vi "Message.vi"(0 "datain":string[](array[string])=["备注", "负载通道", "负载地址", "延时时间", "output max", "output min", "量测类型", "待测物板号"], 5 "HW CH Number":i32, 7 "Setup":string) -> (4 "REPORT INDECATE":string[][](array[string])=[["微安测试", "", "", "", ""], ["微安量测", "4", "0.000", "0.1", "NG"], ["微安量测", "4", "0.000", "0.1", "NG"], ["微安量测", "4", "0.000", "0.1", "NG"], ["微安量测", "4", "0.000", "0.1", "NG"]], 6 "ROW HEAD":string[](array[string]), 8 "PF":string[](array[string]), 10 "testData":string[](array[string]), 15 "Array":string[](array[string]))   [LabVIEW 2018]
panel:
  in  "Bar":bool
  out "结果":bool
  out "Date":string caption="messageBox"
  in  "取消":bool
  in  "确定":bool
  out "数组":bool[](array[boolean])
  # "信息提示！"
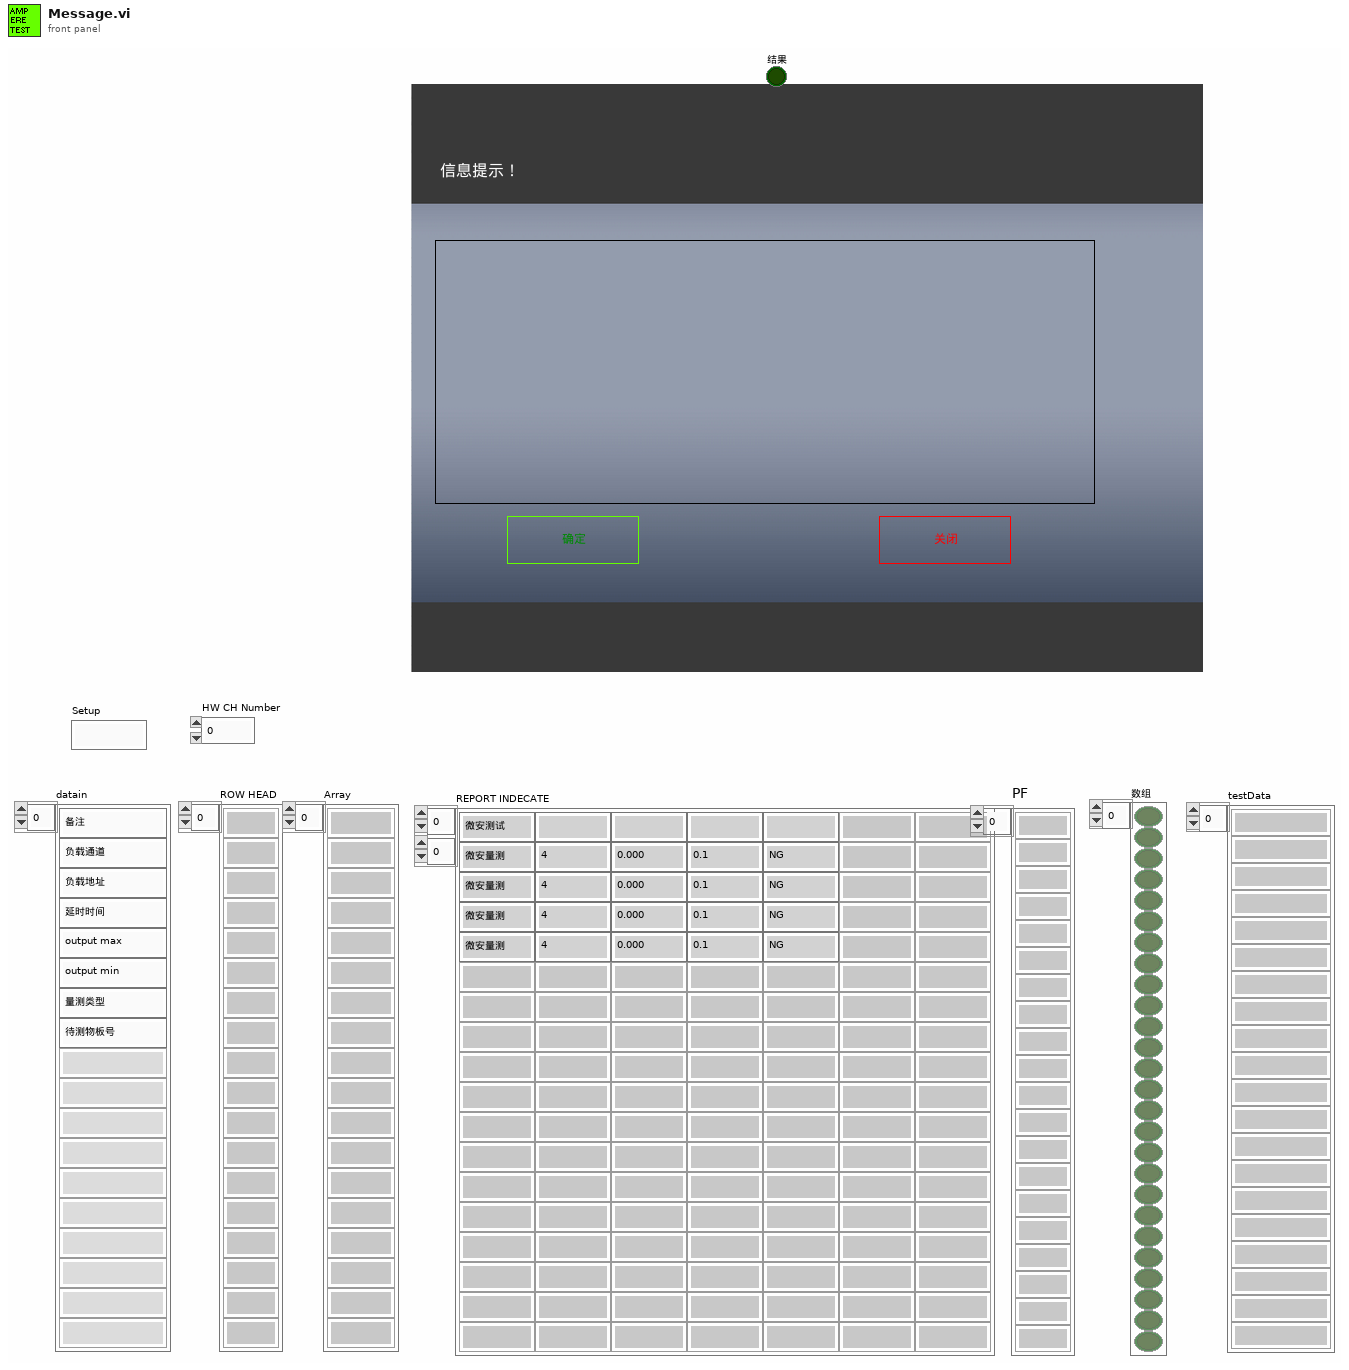
[diagram p1: front panel]
types:
  T1 = typedef "Window Refnum.ctl" = refnum<k1>
  T2 = typedef "Window Rectangle.ctl" = cluster{"left":i16, "top":i16, "right":i16, "bottom":i16}
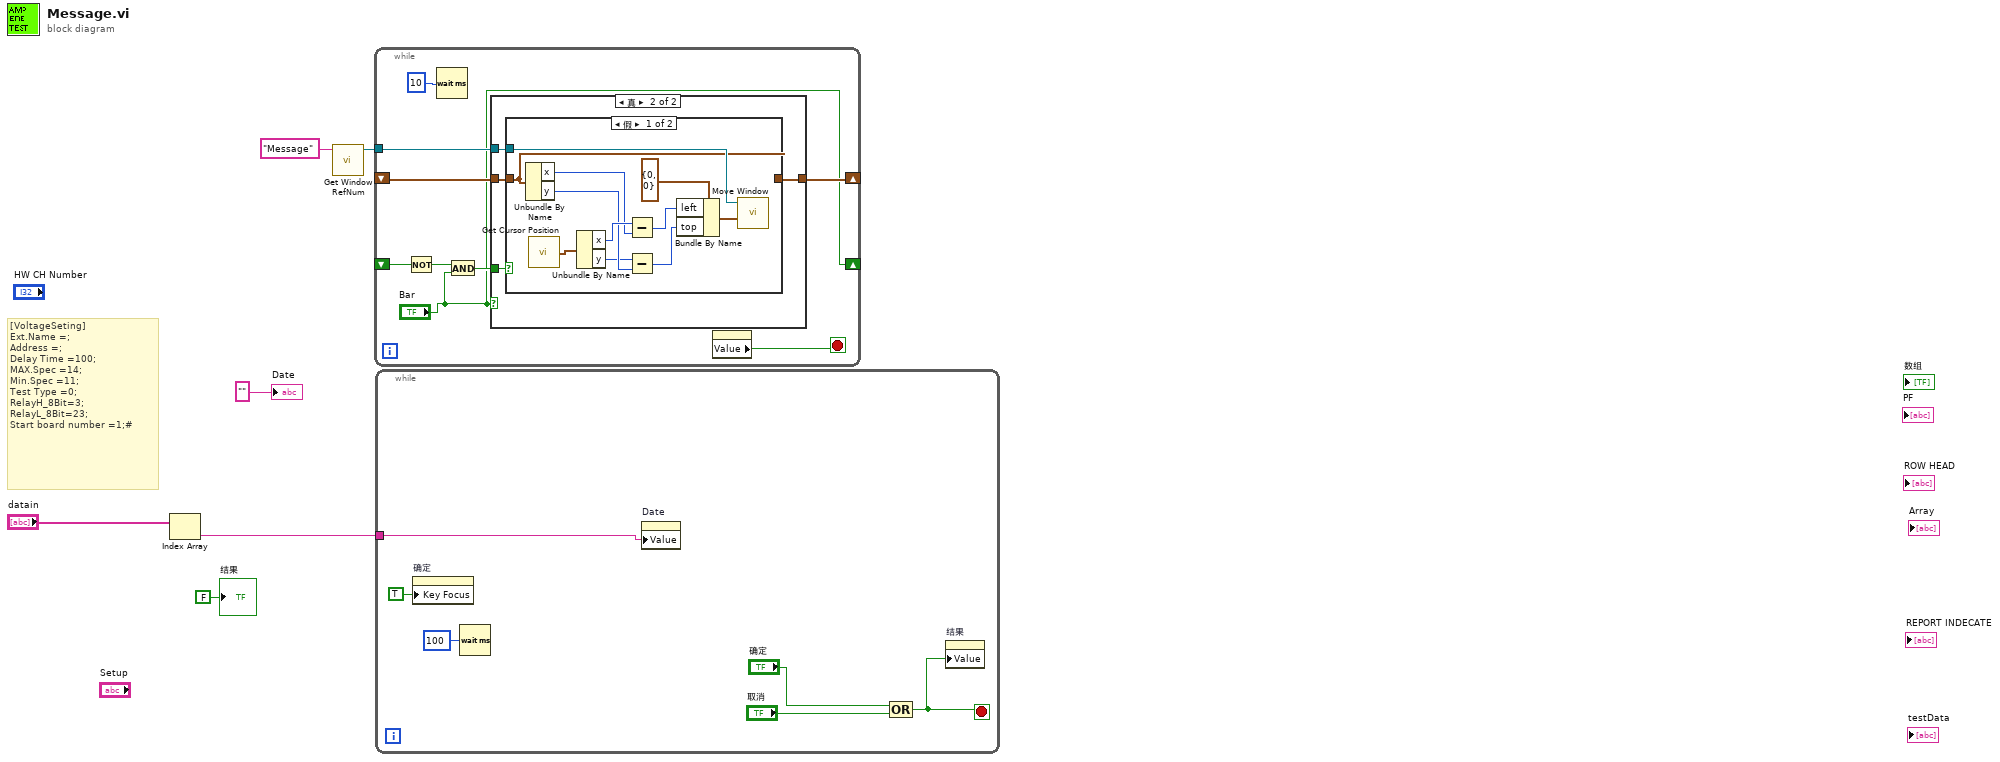
[diagram p0: block diagram]
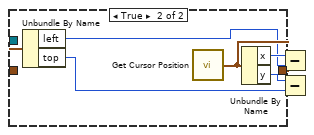
[diagram p3: hidden frame]
diagram:
  # "[VoltageSeting]\nExt.Name =;\nAddress =;\nDelay Time =100;\nMAX.Spec =14;\nMin.Spec =11;\nTest Type =0;\nRelayH_8Bit=3;\nRelayL_8Bit=23;\nStart board number =1;#"
  n1 = Index Array(array="datain") -> (element=w5:string)  [unwired: 1 in]
  n2 = call "Get Window RefNum.vi"("window name (\"\")"="Message" ("window name (\"\")")) -> ("window refnum (NaWR)"=w3:T1)  [unwired: 1 in, 7 out]
  n3 = while {
    shift-left: _ -> [w10]
    shift-right: [w11] -> _
    shift-left: _ -> [w13]
    shift-right: ["Bar"] -> _
    tunnel: w3 -> [w14]
    stop <- w8 stop-if-true
    n4 = Not(x=w13) -> (.not. x?=w12:bool)
    n5 = Wait (ms)(milliseconds to wait=u32 10) -> ()  [unwired: 1 out]
    n6 = And(x=w12, y="Bar") -> (x .and. y?=w9:bool)
    n7 = case shown="真" "Bar" {
      tunnel: w14 -> [_ w20]
      tunnel: [w16 w19] -> w11
      tunnel: w10 -> [w16 w17]
      tunnel: w9 -> [_ w18]
      frame False {
      }
      frame True {
        n8 = case shown="假" w18 {
          tunnel: w20 -> [w26 w42]
          tunnel: [w21 w32] -> w19
          tunnel: w17 -> [w21 _]
          frame False {
            n9 = Unbundle By Name(w21) -> ("x"=w29:i16, "y"=w28:i16)
            n10 = call "Get Cursor Position.vi"() -> ("cursor position"=w31:cluster{"x":i16, "y":i16})
            n11 = Unbundle By Name(w31) -> ("x"=w30:i16, "y"=w27:i16)
            n12 = Subtract(x=w30, y=w29) -> (x-y=w23:i16)
            n13 = Subtract(x=w27, y=w28) -> (x-y=w24:i16)
            n14 = Bundle By Name(cluster=cluster{"left":i16, "top":i16} {"left"=0, "top"=0} ("new position (0,0)"), "left"=w23, "top"=w24) -> (w22:cluster{"left":i16, "top":i16})
            n15 = call "Move Window.vi"("new position (0,0)"=w22, "window refnum (NaWR)"=w26) -> ()  [unwired: 2 in, 4 out]
          }
          frame True {
            n16 = call "Get Window Rectangle.vi"("window refnum (NaWR)"=w42) -> ("window rect"=w41:T2)  [unwired: 1 in, 5 out]
            n17 = call "Extract Window Origin.vi"("window rect"=w41) -> ("window origin"=w40:cluster{"left":i16, "top":i16})  [unwired: 1 out]
            n18 = Unbundle By Name(w40) -> ("left"=w37:i16, "top"=w36:i16)
            n19 = call "Get Cursor Position.vi"() -> ("cursor position"=w39:cluster{"x":i16, "y":i16})
            n20 = Unbundle By Name(w39) -> ("x"=w38:i16, "y"=w35:i16)
            n21 = Subtract(x=w38, y=w37) -> (x-y=w33:i16)
            n22 = Subtract(x=w35, y=w36) -> (x-y=w34:i16)
            n23 = Bundle By Name(cluster=w39, "x"=w33, "y"=w34) -> (w32:cluster{"x":i16, "y":i16})
          }
        }
      }
    }
    n24 = property on="结果" class="Bool (严格)"() -> ("Value"=w8:bool)  [unwired: 2 in, 2 out]
  }
  n25 = while {
    tunnel: w5 -> [w46]
    stop <- w43 stop-if-true
    n26 = property on="确定" class="Bool"("Key Focus"=TRUE ("键选中")) -> ()  [unwired: 2 in, 2 out]
    n27 = Wait (ms)(milliseconds to wait=u32 100 ("等待时间（毫秒）")) -> ()  [unwired: 1 out]
    n28 = property on="Date" class="Str"("Value"=w46) -> ()  [unwired: 2 in, 2 out]
    n29 = Compound Arithmetic op=OR ("复合运算")("确定", "取消") -> (w43:bool)
    n30 = property on="结果" class="Bool (严格)"("Value"=w43) -> ()  [unwired: 2 in, 2 out]
  }
  "Date" <- "" ("Date")
  "结果" <- FALSE ("结果")
